vi "Get FFT - Scaled Spectrums.vi"(0 "reference in":refnum<class "GSwFormDSP.lvclass">, 5 "error in (no error)":errorcluster, 6 "Acoustic Weighting":T1, 7 "Spectrum Display Options":T2, 9 "Spectral Function Type":T3) -> (11 "Spectrum Unit":string[](array[string]), 13 "Scaled Spectrums":waveform(dbl)[](array[waveform]), 14 "reference out":refnum<class "GSwFormDSP.lvclass">, 19 "error out":errorcluster)   [LabVIEW 2020, in "GSwFormDSP.lvclass"]
uses:
  GSwFormDSP.lvclass
  functions/Spectral Function Type.ctl
  functions/Spectrum Display Options.ctl
  functions/Acoustic Weighting.ctl
  <vilib>/Analysis/NI_AALPro.lvlib
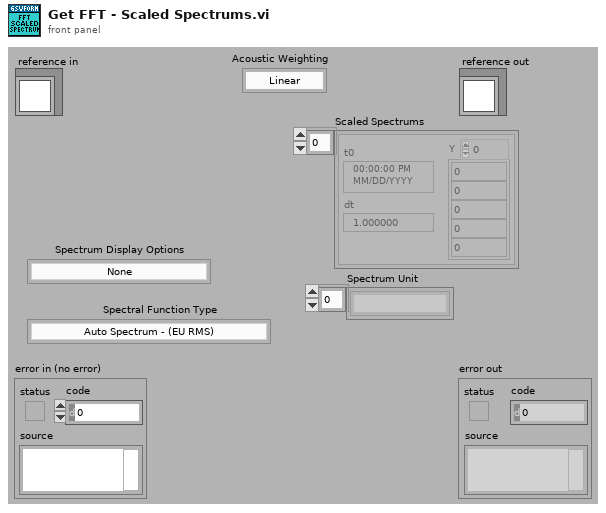
[diagram p1: front panel]
types:
  T1 = typedef "GSwFormDSP.lvclass/Acoustic Weighting.ctl" = enum16{"Linear", "A-weighting"}
  T2 = typedef "GSwFormDSP.lvclass/Spectrum Display Options.ctl" = enum16{"None", "dB - NO reference value", "dB - Automatic reference value", "dB - Sound SPL (ref 20E-6 Pa)", "dB - Acceleration (ref 1E-6 m/s²)", "dB - Velocity (ref 1E-9 m/s)", "dB - Displacement (ref 1E-12 m)"}
  T3 = typedef "GSwFormDSP.lvclass/Spectral Function Type.ctl" = enum16{"Auto Spectrum - (EU RMS)", "Auto Spectrum - (EU Peak)", "Power Spectrum - (EU RMS²)", "Power Spectrum - (EU Peak²)", "Auto Spectrum Density - (EU RMS/rtHz)", "Auto Spectrum Density - (EU Peak/rtHz)", "Power Spectrum Density - (EU RMS²/Hz)", "Power Spectrum Density - (EU Peak²/Hz)"}
  T4 = enum16{"Power (Vrms^2)", "Amplitude (Vrms)", "Gain (amplitude ratio)"}
  T5 = typedef "GSwFormDSP.lvclass/ObjectAttributes.ctl" = cluster{"Wform Ref":refnum<data-value>, "Nb Signals":i32, "Spectral Function Parameters":T6, "FFT":waveform(cdb)[], "Nb FFT":i32, "Nb Averages":i32[], "Reference Indexes":i32[], "Response Indexes":i32[], "Coherence":waveform(dbl)[], "TDF Parameters":T8, "DAQ":cluster{"Duration (sec)":dbl, "Buffer Size (Samples)":i32, "Offset (Samples)":i32}, "Filter Impulse Response (TDF)":waveform(dbl), "Sound Playback":T9}
  T6 = typedef "GSwFormDSP.lvclass/Spectral Parameters.ctl" = cluster{"Frequency resolution (Hz)":dbl, "Overlap":dbl, "Window":T7}
  T7 = typedef "NI_AALPro.lvlib/windowTd.ctl" = u32
  T8 = typedef "GSwFormDSP.lvclass/TDF Parameters.ctl" = cluster{"Filter":enum32{"Lowpass", "Highpass", "Bandpass", "Bandstop"}, "Type:":enum16{"Butterworth", "Chebyshev", "Inv Chebyshev", "Elliptic", "Bessel"}, "LP cutoff freq":dbl, "HP cutoff freq":dbl, "Order":i32, "passband ripple (dB)":dbl, "stopband attenuation (dB)":dbl, "Phaseless Filter":bool, "Include Fade IN and OUT":bool}
  T9 = typedef "GSwFormDSP.lvclass/Sound Playback.ctl" = cluster{"Timer start (ms)":u32, "task ID":T10, "Cursor Init Location (s)":dbl, "SC Volume":dbl}
  T10 = typedef "Sound Output Task ID.ctl" = u32
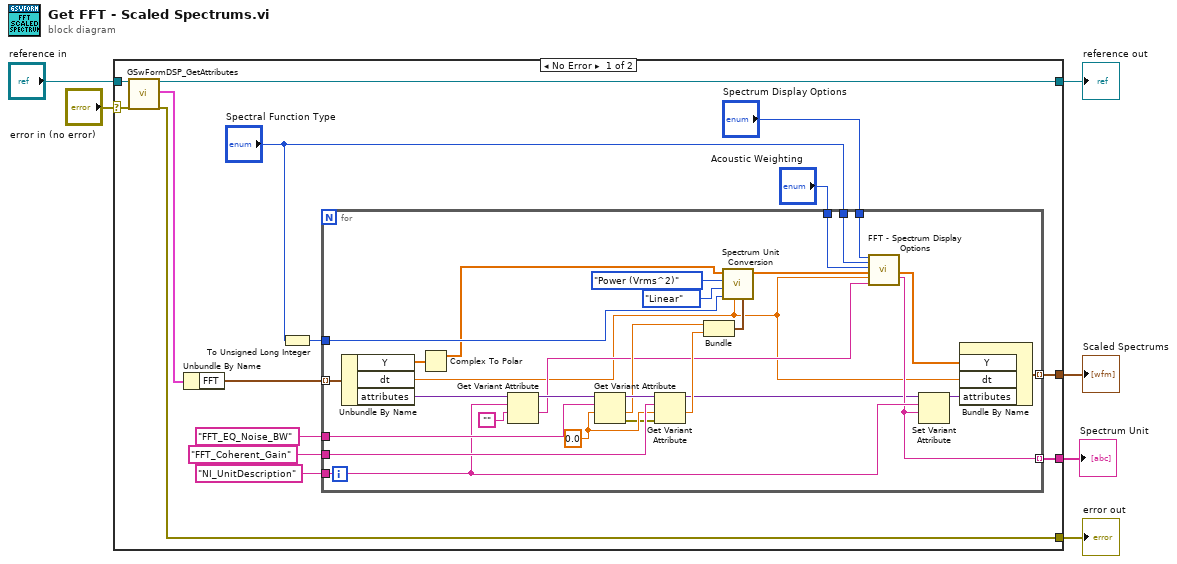
[diagram p0: block diagram]
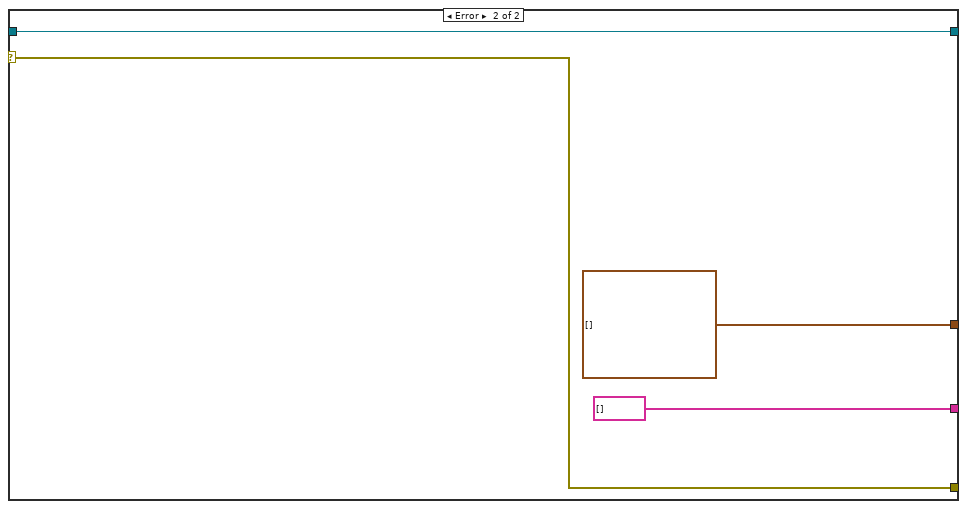
[diagram p2: hidden frame]
diagram:
  n1 = case shown="No Error" "error in (no error)" {
    selector: "error in (no error)" -> [w21 w54]
    tunnel: [w20 w54] -> w5
    tunnel: [w19 w53] -> w3
    tunnel: "reference in" -> [w17 w53]
    tunnel: [w10 waveform(dbl)[] []] -> w2
    tunnel: [w7 string[] []] -> w1
    frame No Error {
      n2 = call "GSwFormDSP_GetAttributes.vi"("reference in"=w17, "error in (no error)"=w21) -> ("reference out"=w19:refnum<class "GSwFormDSP.lvclass">, "attributes"=w18:T5, "error out"=w20:errorcluster)  [unwired: 14 in, 1 out]
      n3 = Unbundle By Name(w18) -> ("FFT"=w11:waveform(cdb)[])
      n4 = To Unsigned Long Integer(number="Spectral Function Type") -> (unsigned 32bit integer=w13:u32)
      n5 = for {
        tunnel: w13 -> [w29]
        tunnel: "FFT_EQ_Noise_BW" ("EQ noise BW (DBL)") -> [w50]
        tunnel: "FFT_Coherent_Gain" ("Coherent Gain (DBL)") -> [w49]
        tunnel: "NI_UnitDescription" ("wform unit") -> [w48]
        tunnel: "Spectrum Display Options" -> [w35]
        tunnel: w11 -> [w47] mode=indexing
        tunnel: [w36] -> w10 mode=indexing
        tunnel: "Acoustic Weighting" -> [w25]
        tunnel: "Spectral Function Type" -> [w34]
        tunnel: [w32] -> w7 mode=indexing
        w42 = 0.0
        n6 = Unbundle By Name(w47) -> ("Y"=w43:cdb[], "dt"=w22:dbl, "attributes"=w31:variant)
        n7 = Complex To Polar(r * e^(i*theta)=w43) -> (r=w28:dbl[])  [unwired: 1 out]
        n8 = Get Variant Attribute(Variant=w31, name=w48, default value (empty Variant)="") -> (duplicate Variant=w30:variant, value=w24:string)  [unwired: 1 in, 2 out]
        n9 = Get Variant Attribute(Variant=w30, name=w50, default value (empty Variant)=w42) -> (duplicate Variant=w41:variant, value=w40:dbl, error out=w38:errorcluster)  [unwired: 1 in, 1 out]
        n10 = Get Variant Attribute(Variant=w41, name=w49, default value (empty Variant)=w42, error in=w38) -> (duplicate Variant=w26:variant, value=w39:dbl)  [unwired: 2 out]
        n11 = Bundle(w40, w39) -> (w44:cluster{dbl, dbl})  [unwired: 1 out]
        n12 = call <vilib>:"Spectrum Unit Conversion.vi"("window constants"=w44, "df"=w22, "display unit"=w29, "log/linear"=enum16{"Linear", "dB", "dBm"}."Linear", "spectrum type"=T4."Power (Vrms^2)", "Spectrum in"=w28) -> ("Spectrum out"=w27:dbl[])  [unwired: 1 in, 4 out]
        n13 = call "FFT - Spectrum Display Options.vi"("Spectrum Display Options"=w35, "Spectral Function Type"=w34, "Acoustic Weighting"=w25, "Spectrum Mag IN"=w27, "dF (Hz)"=w22, "Unit IN"=w24) -> ("Spectrum Mag OUT"=w33:dbl[], "Unit OUT"=w32:string)  [unwired: 12 in]
        n14 = Set Variant Attribute(Variant=w26, name=w48, value=w32) -> (Variant out=w23:variant)  [unwired: 1 in, 2 out]
        n15 = Bundle By Name("Y"=w33, "dt"=w22, "attributes"=w23) -> (w36:waveform(dbl))  [unwired: 1 in]
      }
    }
    frame Error {
    }
  }
  "error out" <- w5
  "reference out" <- w3
  "Scaled Spectrums" <- w2
  "Spectrum Unit" <- w1
